vi "Format Sweep AO AI.vi"(6 "Sweeping?":bool, 7 "ChassisSerialNumber":u32, 9 "Channel":i32, 11 "waveform":waveform(dbl)) -> (2 "Times":timestamp[](array[timestamp]), 3 "Log Data":T1[](array[typedef]))   [LabVIEW 2019, in "Instrument.Lockin.lvlib" / "Instrument.Lockin.lvclass"]
uses:
  Instrument.Lockin.lvclass
  Typedefs/Lockin.LogSweepAOAI--Cluster.ctl
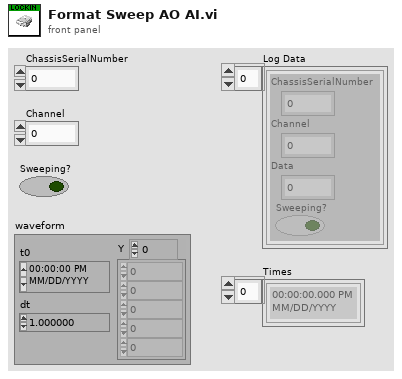
[diagram p1: front panel]
types:
  T1 = typedef "Instrument.Lockin.lvlib/Instrument.Lockin.lvclass/Lockin.LogSweepAOAI--Cluster.ctl" = cluster{"ChassisSerialNumber":u32, "Channel":i32, "Data":dbl, "Sweeping?":bool}
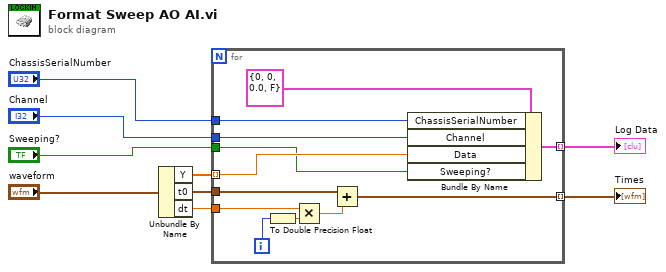
[diagram p0: block diagram]
diagram:
  n1 = Unbundle By Name("waveform") -> ("Y"=w3:dbl[], "t0"=w1:timestamp, "dt"=w2:dbl)
  n2 = for {
    tunnel: w1 -> [w17]
    tunnel: w2 -> [w21]
    tunnel: [w16] -> w9 mode=indexing
    tunnel: w3 -> [w14] mode=indexing
    tunnel: "ChassisSerialNumber" -> [w13]
    tunnel: "Channel" -> [w12]
    tunnel: "Sweeping?" -> [w11]
    tunnel: [w10] -> w8 mode=indexing
    i -> [w20]
    n3 = To Double Precision Float(number=w20) -> (double precision float=w19:dbl)
    n4 = Multiply(x=w21, y=w19) -> (x*y=w18:dbl)
    n5 = Add(x=w17, y=w18) -> (x+y=w16:timestamp)
    n6 = Bundle By Name(cluster=T1 {"ChassisSerialNumber"=0, "Channel"=0, "Data"=0.0, "Sweeping?"=FALSE}, "ChassisSerialNumber"=w13, "Channel"=w12, "Data"=w14, "Sweeping?"=w11) -> (w10:T1)
  }
  "Times" <- w9
  "Log Data" <- w8
